vi "WaveformChartGraph.vi"() -> ()   [LabVIEW 2018]
panel:
  out "Array":dbl[](array[numeric])
  out "Waveform Graph":dbl[](graph)
  out "Waveform Chart":dbl(graph)
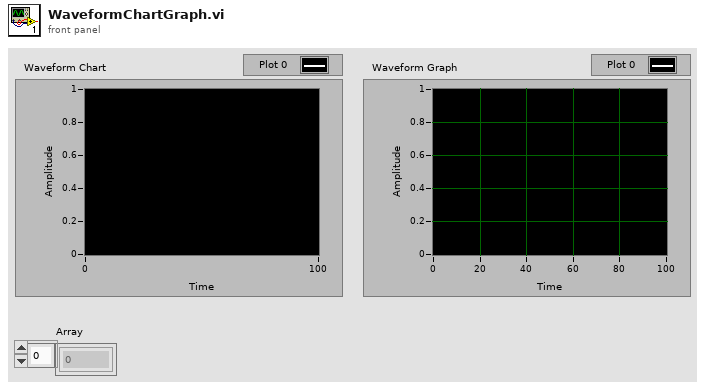
[diagram p1: front panel]
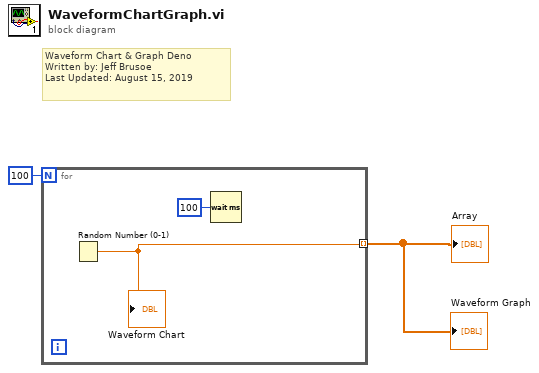
[diagram p0: block diagram]
diagram:
  # "Waveform Chart & Graph Deno\nWritten by: Jeff Brusoe\nLast Updated: August 15, 2019"
  n1 = for {
    N: 100 -> [_]
    tunnel: [w4] -> w1 mode=indexing
    n2 = Random Number (0-1)() -> (number: 0 to 1=w4:dbl)
    "Waveform Chart" <- w4
    n3 = Wait (ms)(milliseconds to wait=u32 100) -> ()  [unwired: 1 out]
  }
  "Waveform Graph" <- w1
  "Array" <- w1
